vi "Acquire_Path_Relation.vi"(10 "Topology Matrix":dbl[][](array[numeric])=[[1.0, 1.0, 0.0], [1.0, 0.0, 1.0]]) -> (2 "Path Relation topology":dbl[][](array[numeric]))   [LabVIEW 2014]
doc: "拓扑矩阵描述节点的相邻关系"
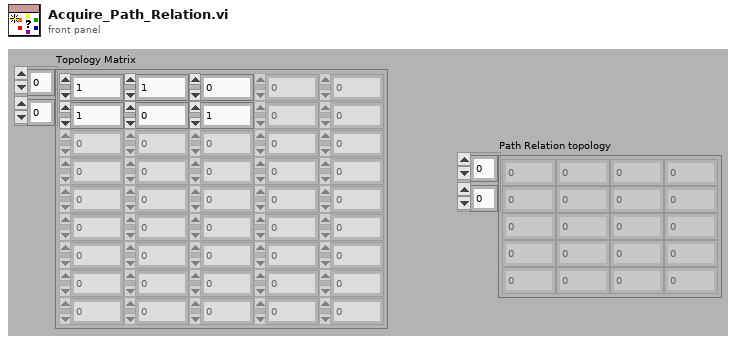
[diagram p1: front panel]
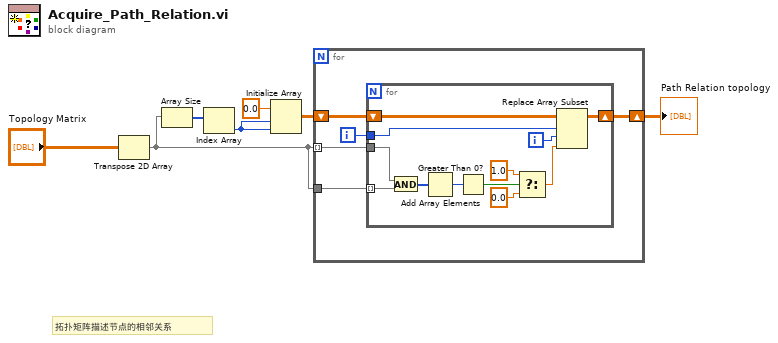
[diagram p0: block diagram]
diagram:
  # "拓扑矩阵描述节点的相邻关系"
  n1 = Transpose 2D Array(2D array="Topology Matrix") -> (transposed array=w1:dbl[][])
  n2 = Array Size(array=w1) -> (size(s)=w7:i32[])
  n3 = Index Array(array=w7) -> (element=w5:i32)  [unwired: 1 in]
  n4 = Initialize Array(0.0 ("元素"), w5, w5) -> (w4:dbl[][])
  n5 = for {
    tunnel: w1 -> [w12] mode=indexing
    tunnel: w1 -> [w11]
    shift-right: [w9] -> w3
    shift-left: w4 -> [w10]
    i -> [w8]
    n6 = for {
      tunnel: w12 -> [w24]
      tunnel: w11 -> [w23] mode=indexing
      shift-right: [w19] -> w9
      shift-left: w10 -> [w22]
      tunnel: w8 -> [w21]
      i -> [w20]
      n7 = And(x=w24, y=w23) -> (x .and. y?=w18:i32[])
      n8 = Add Array Elements(numeric array=w18) -> (sum=w17:i32)
      n9 = Greater Than 0?(x=w17) -> (x > 0?=w16:bool)
      n10 = Select(t=1.0, s=w16, f=0.0) -> (s? t:f=w13:dbl)
      n11 = Replace Array Subset(array=w22, new element=w13, index (row)=w21, index (col)=w20) -> (w19:dbl[][])
    }
  }
  "Path Relation topology" <- w3
